vi "Error handler log.vi"(0 "input":string, 1 "error source VI":path, 3 "error in":errorcluster, 4 "clear error":bool=TRUE, 5 "auto detect":bool=TRUE) -> (7 "log":string="2:40 PM\tStop DAQ...", 10 "error out":errorcluster)   [LabVIEW 2024]
panel:
  out "error log file":path
  in  "platform":u16
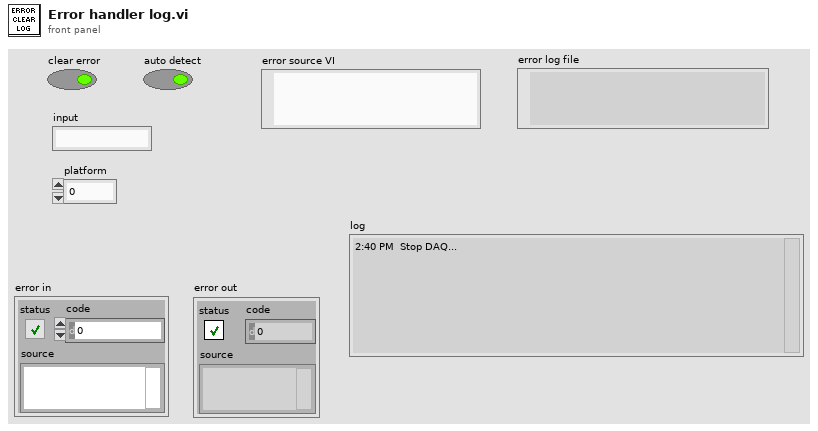
[diagram p1: front panel]
types:
  T1 = enum16{"open", "replace", "create", "open or create", "replace or create", "replace or create with confirmation"}
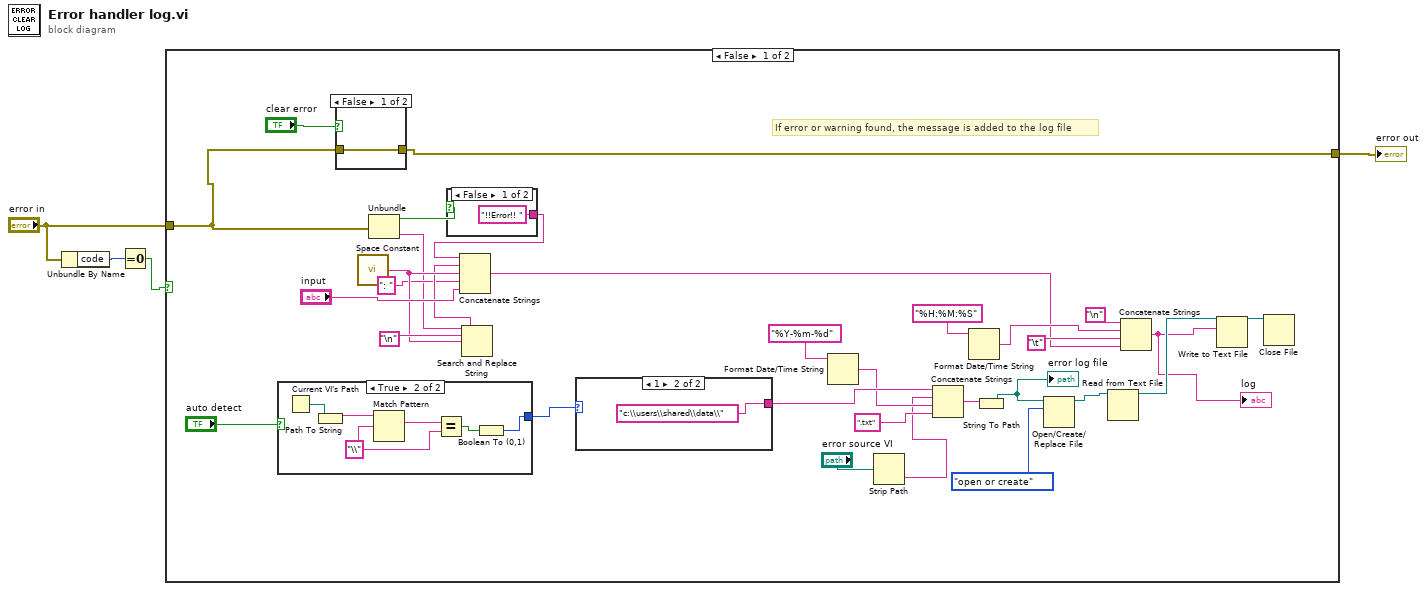
[diagram p0: block diagram]
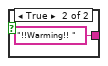
[diagram p2: hidden frame]
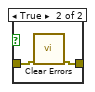
[diagram p3: hidden frame]
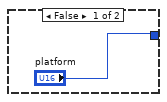
[diagram p4: hidden frame]
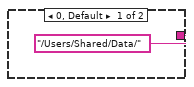
[diagram p5: hidden frame]
diagram:
  n1 = Unbundle By Name("error in") -> ("code"=w4:i32)
  n2 = Equal To 0?(x=w4) -> (x = 0?=w2:bool)
  n3 = case shown="False" w2 {
    tunnel: "error in" -> [w17 w50]
    tunnel: [w9 w50] -> w1
    frame False {
      # "If error or warning found, the message is added to the log file"
      n4 = case shown="True" "auto detect" {
        tunnel: ["platform" w42] -> w18
        frame False {
        }
        frame True {
          w46 = "\\" ("regular expression")
          n5 = Current VI's Path() -> (path=w43:path)
          n6 = Path To String(path=w43) -> (string=w45:string)
          n7 = Match Pattern(string=w45, regular expression=w46) -> (match substring=w47:string)  [unwired: 4 out]
          n8 = Equal?(x=w47, y=w46) -> (x = y?=w44:bool)
          n9 = Boolean To (0,1)(Boolean=w44) -> (0, 1=w42:i16)
        }
      }
      n10 = case shown="False" "clear error" {
        tunnel: w17 -> [w38 w40]
        tunnel: [w38 w39] -> w9
        frame False {
        }
        frame True {
          n11 = call <vilib>:"Clear Errors.vi"("error in (no error)"=w40) -> ("error out"=w39:errorcluster)  [unwired: 5 in, 1 out]
        }
      }
      n12 = call <vilib>:"Space Constant.vi"() -> ("String"=w12:string)
      n13 = Unbundle(w17) -> ("status"=w15:bool, "source"=w8:string)  [unwired: 1 out]
      n14 = case shown="False" w15 {
        tunnel: ["!!Error!! " ("string") "!!Warming!! " ("string")] -> w14
        frame False {
        }
        frame True {
        }
      }
      n15 = Search and Replace String(input string=w8, search string="\n", replace string=w12) -> (result string=w11:string)  [unwired: 5 in, 3 out]
      n16 = Concatenate Strings(w14, w11, w12, ": " ("string"), "input") -> (w20:string)
      n17 = case shown="1" w18 {
        tunnel: ["/Users/Shared/Data/" ("string") "c:\\users\\shared\\data\\" ("string")] -> w26
        frame 0, Default {
        }
        frame 1 {
        }
      }
      n18 = Format Date/Time String(time format string (%c)="%Y-%m-%d") -> (date/time string=w24:string)  [unwired: 2 in]
      n19 = Strip Path(path="error source VI") -> (name=w5:string)  [unwired: 1 out]
      n20 = Concatenate Strings(w26, w5, w24, ".txt" ("string")) -> (w27:string)
      n21 = Format Date/Time String(time format string (%c)="%H:%M:%S") -> (date/time string=w35:string)  [unwired: 2 in]
      n22 = String To Path(string=w27) -> (path=w31:path)
      "error log file" <- w31
      n23 = Open/Create/Replace File(file path (use dialog)=w31, operation (0:open)=T1."open or create") -> (refnum out=w33:refnum<file>)  [unwired: 4 in, 2 out]
      n24 = Read from Text File(file (use dialog)=w33) -> (refnum out=w30:refnum<file>)  [unwired: 3 in, 3 out]
      n25 = Concatenate Strings("\n", w35, "\t", w20) -> (w7:string)
      "log" <- w7
      n26 = Write to Text File(file (use dialog)=w30, text=w7) -> (refnum out=w34:refnum<file>)  [unwired: 2 in, 2 out]
      n27 = Close File(refnum=w34) -> ()  [unwired: 1 in, 2 out]
    }
    frame True {
    }
  }
  "error out" <- w1
